vi "HandleObservationSync.vi"(8 "error in (no error)":errorcluster, 11 "S4GUI in":refnum<class "S4GUI.lvclass">) -> (0 "error out":errorcluster, 3 "S4GUI out":refnum<class "S4GUI.lvclass">)   [LabVIEW 2018, in "S4GUI.lvclass"] (continued)
              n761 = call-dynamic "Write Channel.vi"("error in (no error)"=w2070, "Channel.lvclass"=w2072, "Acquisition in"=w2077) -> ("error out"=w2075:errorcluster, "Acquisition out"=w2076:refnum<class "Acquisition.lvclass">)  [unwired: 7 in]
            }
          }
          n762 = call-dynamic "Write AcquisitionA.vi"("error in (no error)"=w1986, "Acquisition.lvclass"=w1988, "S4ACS_GUI in"=w1987) -> ("error out"=w1982:errorcluster, "S4ACS_GUI out"=w1981:refnum<class "S4GUI.lvclass">)  [unwired: 7 in]
          n763 = call "Read AcquisitionB.vi"("error in (no error)"=w1982, "S4ACS_GUI in"=w1981) -> ("error out"=w1964:errorcluster, "Acquisition.lvclass"=w1967:refnum<class "Acquisition.lvclass">, "S4ACS_GUI out"=w1968:refnum<class "S4GUI.lvclass">)  [unwired: 7 in]
          n764 = call "Read connection.vi"("error in (no error)"=w1964, "Server in"=w1967) -> ("error out"=w1963:errorcluster, "connection"=w1965:bool, "Server out"=w1966:refnum<class "Acquisition.lvclass">)  [unwired: 7 in]
          n765 = case shown="True" w1965 {
            tunnel: w1966 -> [w2045 w2061]
            tunnel: w1963 -> [w2044 w2060]
            tunnel: [w2045 w2058] -> w1962
            tunnel: [w2044 w2057] -> w1961
            tunnel: [0 ("State") w2047] -> w1931
            frame False {
            }
            frame True {
              n766 = call-dynamic "Read Channel.vi"("error in (no error)"=w2060, "Acquisition in"=w2061) -> ("error out"=w2056:errorcluster, "Channel.lvclass"=w2055:refnum<class "Channel.lvclass">, "Acquisition out"=w2059:refnum<class "Acquisition.lvclass">)  [unwired: 7 in]
              n767 = call-dynamic "Read State Machine.vi"("error in (no error)"=w2056, "Device in"=w2055) -> ("error out"=w2049:errorcluster, "State Machine.lvclass"=w2051:refnum<class "State Machine.lvclass">, "Device out"=w2053:refnum<class "Channel.lvclass">)  [unwired: 7 in]
              n768 = call-dynamic "Read State.vi"("error in (no error)"=w2049, "State Machine in"=w2051) -> ("error out"=w2048:errorcluster, "State"=w2047:i32, "State Machine out"=w2050:refnum<class "State Machine.lvclass">)  [unwired: 7 in]
              n769 = call-dynamic "Write State Machine.vi"("error in (no error)"=w2048, "State Machine.lvclass"=w2050, "Device in"=w2053) -> ("error out"=w2052:errorcluster, "Device out"=w2054:refnum<class "Channel.lvclass">)  [unwired: 7 in]
              n770 = call-dynamic "Write Channel.vi"("error in (no error)"=w2052, "Channel.lvclass"=w2054, "Acquisition in"=w2059) -> ("error out"=w2057:errorcluster, "Acquisition out"=w2058:refnum<class "Acquisition.lvclass">)  [unwired: 7 in]
            }
          }
          n771 = call "Write AcquisitionB.vi"("error in (no error)"=w1961, "Acquisition.lvclass"=w1962, "S4ACS_GUI in"=w1968) -> ("error out"=w1980:errorcluster, "S4ACS_GUI out"=w1979:refnum<class "S4GUI.lvclass">)  [unwired: 7 in]
          n772 = call-dynamic "Read AcquisitionC.vi"("error in (no error)"=w1980, "S4ACS_GUI in"=w1979) -> ("error out"=w1959:errorcluster, "Acquisition.lvclass"=w1960:refnum<class "Acquisition.lvclass">, "S4ACS_GUI out"=w1984:refnum<class "S4GUI.lvclass">)  [unwired: 7 in]
          n773 = call "Read connection.vi"("error in (no error)"=w1959, "Server in"=w1960) -> ("error out"=w1958:errorcluster, "connection"=w1956:bool, "Server out"=w1957:refnum<class "Acquisition.lvclass">)  [unwired: 7 in]
          n774 = case shown="True" w1956 {
            tunnel: w1957 -> [w2027 w2043]
            tunnel: w1958 -> [w2026 w2042]
            tunnel: [w2027 w2040] -> w1955
            tunnel: [w2026 w2039] -> w1954
            tunnel: [0 ("State") w2029] -> w1930
            frame False {
            }
            frame True {
              n775 = call-dynamic "Read Channel.vi"("error in (no error)"=w2042, "Acquisition in"=w2043) -> ("error out"=w2038:errorcluster, "Channel.lvclass"=w2037:refnum<class "Channel.lvclass">, "Acquisition out"=w2041:refnum<class "Acquisition.lvclass">)  [unwired: 7 in]
              n776 = call-dynamic "Read State Machine.vi"("error in (no error)"=w2038, "Device in"=w2037) -> ("error out"=w2031:errorcluster, "State Machine.lvclass"=w2033:refnum<class "State Machine.lvclass">, "Device out"=w2035:refnum<class "Channel.lvclass">)  [unwired: 7 in]
              n777 = call-dynamic "Read State.vi"("error in (no error)"=w2031, "State Machine in"=w2033) -> ("error out"=w2030:errorcluster, "State"=w2029:i32, "State Machine out"=w2032:refnum<class "State Machine.lvclass">)  [unwired: 7 in]
              n778 = call-dynamic "Write State Machine.vi"("error in (no error)"=w2030, "State Machine.lvclass"=w2032, "Device in"=w2035) -> ("error out"=w2034:errorcluster, "Device out"=w2036:refnum<class "Channel.lvclass">)  [unwired: 7 in]
              n779 = call-dynamic "Write Channel.vi"("error in (no error)"=w2034, "Channel.lvclass"=w2036, "Acquisition in"=w2041) -> ("error out"=w2039:errorcluster, "Acquisition out"=w2040:refnum<class "Acquisition.lvclass">)  [unwired: 7 in]
            }
          }
          n780 = call-dynamic "Write AcquisitionC.vi"("error in (no error)"=w1954, "Acquisition.lvclass"=w1955, "S4ACS_GUI in"=w1984) -> ("error out"=w1978:errorcluster, "S4ACS_GUI out"=w1977:refnum<class "S4GUI.lvclass">)  [unwired: 7 in]
          n781 = call-dynamic "Read AcquisitionD.vi"("error in (no error)"=w1978, "S4ACS_GUI in"=w1977) -> ("error out"=w1951:errorcluster, "Acquisition.lvclass"=w1953:refnum<class "Acquisition.lvclass">, "S4ACS_GUI out"=w1983:refnum<class "S4GUI.lvclass">)  [unwired: 7 in]
          n782 = call "Read connection.vi"("error in (no error)"=w1951, "Server in"=w1953) -> ("error out"=w1950:errorcluster, "connection"=w1949:bool, "Server out"=w1952:refnum<class "Acquisition.lvclass">)  [unwired: 7 in]
          n783 = case shown="True" w1949 {
            tunnel: w1952 -> [w2009 w2025]
            tunnel: w1950 -> [w2008 w2024]
            tunnel: [w2009 w2022] -> w1948
            tunnel: [w2008 w2021] -> w1947
            tunnel: [0 ("State") w2011] -> w1929
            frame False {
            }
            frame True {
              n784 = call-dynamic "Read Channel.vi"("error in (no error)"=w2024, "Acquisition in"=w2025) -> ("error out"=w2020:errorcluster, "Channel.lvclass"=w2019:refnum<class "Channel.lvclass">, "Acquisition out"=w2023:refnum<class "Acquisition.lvclass">)  [unwired: 7 in]
              n785 = call-dynamic "Read State Machine.vi"("error in (no error)"=w2020, "Device in"=w2019) -> ("error out"=w2013:errorcluster, "State Machine.lvclass"=w2015:refnum<class "State Machine.lvclass">, "Device out"=w2017:refnum<class "Channel.lvclass">)  [unwired: 7 in]
              n786 = call-dynamic "Read State.vi"("error in (no error)"=w2013, "State Machine in"=w2015) -> ("error out"=w2012:errorcluster, "State"=w2011:i32, "State Machine out"=w2014:refnum<class "State Machine.lvclass">)  [unwired: 7 in]
              n787 = call-dynamic "Write State Machine.vi"("error in (no error)"=w2012, "State Machine.lvclass"=w2014, "Device in"=w2017) -> ("error out"=w2016:errorcluster, "Device out"=w2018:refnum<class "Channel.lvclass">)  [unwired: 7 in]
              n788 = call-dynamic "Write Channel.vi"("error in (no error)"=w2016, "Channel.lvclass"=w2018, "Acquisition in"=w2023) -> ("error out"=w2021:errorcluster, "Acquisition out"=w2022:refnum<class "Acquisition.lvclass">)  [unwired: 7 in]
            }
          }
          n789 = call-dynamic "Write AcquisitionD.vi"("error in (no error)"=w1947, "Acquisition.lvclass"=w1948, "S4ACS_GUI in"=w1983) -> ("error out"=w1976:errorcluster, "S4ACS_GUI out"=w1941:refnum<class "S4GUI.lvclass">)  [unwired: 7 in]
          n790 = Equal?(x=w1933, y=w1932) -> (x = y?=w1937:bool)
          n791 = Equal?(x=w1942, y=w1932) -> (x = y?=w1946:bool)
          n792 = Equal?(x=w1933, y=w1931) -> (x = y?=w1936:bool)
          n793 = Equal?(x=w1942, y=w1931) -> (x = y?=w1945:bool)
          n794 = Equal?(x=w1933, y=w1930) -> (x = y?=w1935:bool)
          n795 = Equal?(x=w1942, y=w1930) -> (x = y?=w1944:bool)
          n796 = Equal?(x=w1933, y=w1929) -> (x = y?=w1934:bool)
          n797 = Equal?(x=w1942, y=w1929) -> (x = y?=w1943:bool)
          n798 = Compound Arithmetic op=ADD(w1932, w1931, w1930, w1929) -> (w1940:i32)
          n799 = Compound Arithmetic op=OR(w1937, w1936, w1935, w1934) -> (w1927:bool)
          n800 = Compound Arithmetic op=OR(w1946, w1945, w1944, w1943) -> (w1928:bool)
          n801 = Build Array(w1928, w1927) -> (w1926:bool[])
          n802 = Boolean Array To Number(Boolean array=w1926) -> (number=w1925:u32)
          n803 = case shown="0, Default" w1925 {
            tunnel: w1941 -> [w1991 w1999 w2003 w2007]
            tunnel: [w1990 w1998 w2002 w2006] -> w1938
            tunnel: w1940 -> [w1995 _ _ _]
            tunnel: w1939 -> [w1992 _ _ _]
            frame 0, Default {
              n804 = Equal To 0?(x=w1995) -> (x = 0?=w1994:bool)
              n805 = Select(t=u32 360, s=w1994, f=w1992) -> (s? t:f=w1989:u32)
              n806 = Bundle By Name(cluster=w1991, "Obs_state"=w1989) -> (w1990:refnum<class "S4GUI.lvclass">)
            }
            frame 1 {
              n807 = Bundle By Name(cluster=w1999, "Obs_state"=u32 1, "Error Msg"="ERROR: Some channel initialization failed. S4GUI:HandleObservationSync.vi state 272.") -> (w1998:refnum<class "S4GUI.lvclass">)
            }
            frame 2 {
              n808 = Bundle By Name(cluster=w2003, "Obs_state"=u32 1, "Error Msg"="ERROR: Some channel with invalid Exposition Time. S4GUI:HandleObservationSync.vi state 272.") -> (w2002:refnum<class "S4GUI.lvclass">)
            }
            frame 3 {
              n809 = Bundle By Name(cluster=w2007, "Obs_state"=u32 1, "Error Msg"="ERROR: Invalid configuration in the channels. S4GUI:HandleObservationSync.vi state 272.") -> (w2006:refnum<class "S4GUI.lvclass">)
            }
          }
        }
        frame 299 {
          # "Verifcando iniciação dos CICLO:"
          # "T= todos os canais ativos estão zerados."
          # "Exemplo de erro em \"Cycles_done\":\nchA; cycles_done=0; CCD_STATUS=ACTIVE;                                           Seqs_done=15;\nchA; cycles_done=0; CCD_STATUS=IDLE;                                                Seqs_done=16;   =>mudança de seq. com mesmo ciclo\nchA; cycles_done=1; CCD_STATUS=WAITING_EXPOSE_COMMAND; Seqs_done=0;\n\nchB; cycles_done=0; CCD_STATUS=ACTIVE;                                           Seqs_done=15;\nchB; cycles_done=1; CCD_STATUS=WAITING_EXPOSE_COMMAND; Seqs_done=0;     => mudança de seq com novo ciclo"
          # "T=canais receberam STOP"
          # "T= Todos os canais ativos no mesmo ciclo;\nF= Canais em ciclo diferente."
          # "Todos os CYCLES_DONE \nestão zerados?\nSe sim, vai para 327."
          # "Exemplo:\nSET #CYCLES 3\nSET #SEQ 4\ntotal de sequencias: 3 x 4 = 12\n\nseq.        CYCLES_DONE           SEQS_DONE\n1a.                     0                                 0\n2a.                     0                                 1 \n3a.                     0                                 2 \n4a.                     0                                 3 \n                          1                                 4\n5a.                     1                                 0 \n6a.                     1                                 1 \n7a.                     1                                 2 \n8a.                     1                                 3 \n                          2                                 4\n9a.                     2                                 0 \n10a.                   2                                 1 \n11a.                   2                                 2 \n12a.                   2                                 3 \n\nfim                    3                                 4"
          n810 = call-dynamic "Read AcquisitionA.vi"("error in (no error)"=w2132, "S4ACS_GUI in"=w2098) -> ("error out"=w2113:errorcluster, "Acquisition.lvclass"=w2114:refnum<class "Acquisition.lvclass">, "S4ACS_GUI out"=w2134:refnum<class "S4GUI.lvclass">)  [unwired: 7 in]
          n811 = call-dynamic "Read enabled.vi"("error in (no error)"=w2113, "Server in"=w2114) -> ("error out"=w2112:errorcluster, "enabled"=w2093:bool, "Server out"=w2111:refnum<class "Acquisition.lvclass">)  [unwired: 7 in]
          n812 = case shown="True" w2093 {
            tunnel: w2112 -> [w2224 w2240]
            tunnel: [w2225 w2238] -> w2135
            tunnel: [w2224 w2237] -> w2133
            tunnel: [u32 0 ("SequesDone") w2236] -> _
            tunnel: w2111 -> [w2225 w2235]
            tunnel: [TRUE w2234] -> w2097
            tunnel: [FALSE ("stopping") w2227] -> w2089
            frame False {
            }
            frame True {
              # "CYCLES_DONE = 0 ?"
              n813 = call-dynamic "Read Channel.vi"("error in (no error)"=w2240, "Acquisition in"=w2235) -> ("error out"=w2232:errorcluster, "Channel.lvclass"=w2233:refnum<class "Channel.lvclass">, "Acquisition out"=w2239:refnum<class "Acquisition.lvclass">)  [unwired: 7 in]
              n814 = call-dynamic "Read CyclesDone.vi"("error in (no error)"=w2232, "Channel in"=w2233) -> ("error out"=w2230:errorcluster, "CyclesDone"=w2236:u32, "Channel out"=w2231:refnum<class "Channel.lvclass">)  [unwired: 7 in]
              n815 = Equal?(x=w2236, y=u32 0) -> (x = y?=w2234:bool)
              n816 = call-dynamic "Read stopping.vi"("error in (no error)"=w2230, "Channel in"=w2231) -> ("error out"=w2229:errorcluster, "stopping"=w2227:bool, "Channel out"=w2228:refnum<class "Channel.lvclass">)  [unwired: 7 in]
              n817 = call-dynamic "Write Channel.vi"("error in (no error)"=w2229, "Channel.lvclass"=w2228, "Acquisition in"=w2239) -> ("error out"=w2237:errorcluster, "Acquisition out"=w2238:refnum<class "Acquisition.lvclass">)  [unwired: 7 in]
            }
          }
          n818 = call-dynamic "Write AcquisitionA.vi"("error in (no error)"=w2133, "Acquisition.lvclass"=w2135, "S4ACS_GUI in"=w2134) -> ("error out"=w2130:errorcluster, "S4ACS_GUI out"=w2129:refnum<class "S4GUI.lvclass">)  [unwired: 7 in]
          n819 = call "Read AcquisitionB.vi"("error in (no error)"=w2130, "S4ACS_GUI in"=w2129) -> ("error out"=w2107:errorcluster, "Acquisition.lvclass"=w2110:refnum<class "Acquisition.lvclass">, "S4ACS_GUI out"=w2131:refnum<class "S4GUI.lvclass">)  [unwired: 7 in]
          n820 = call-dynamic "Read enabled.vi"("error in (no error)"=w2107, "Server in"=w2110) -> ("error out"=w2108:errorcluster, "enabled"=w2092:bool, "Server out"=w2109:refnum<class "Acquisition.lvclass">)  [unwired: 7 in]
          n821 = case shown="True" w2092 {
            tunnel: w2108 -> [w2204 w2220]
            tunnel: w2109 -> [w2205 w2219]
            tunnel: [u32 0 ("SequesDone") w2214] -> _
            tunnel: [w2204 w2218] -> w2128
            tunnel: [w2205 w2217] -> w2127
            tunnel: [TRUE w2213] -> w2096
            tunnel: [FALSE ("stopping") w2207] -> w2088
            frame False {
            }
            frame True {
              n822 = call-dynamic "Read Channel.vi"("error in (no error)"=w2220, "Acquisition in"=w2219) -> ("error out"=w2211:errorcluster, "Channel.lvclass"=w2212:refnum<class "Channel.lvclass">, "Acquisition out"=w2215:refnum<class "Acquisition.lvclass">)  [unwired: 7 in]
              n823 = call-dynamic "Read CyclesDone.vi"("error in (no error)"=w2211, "Channel in"=w2212) -> ("error out"=w2209:errorcluster, "CyclesDone"=w2214:u32, "Channel out"=w2216:refnum<class "Channel.lvclass">)  [unwired: 7 in]
              n824 = Equal?(x=w2214, y=u32 0) -> (x = y?=w2213:bool)
              n825 = call-dynamic "Read stopping.vi"("error in (no error)"=w2209, "Channel in"=w2216) -> ("error out"=w2208:errorcluster, "stopping"=w2207:bool, "Channel out"=w2210:refnum<class "Channel.lvclass">)  [unwired: 7 in]
              n826 = call-dynamic "Write Channel.vi"("error in (no error)"=w2208, "Channel.lvclass"=w2210, "Acquisition in"=w2215) -> ("error out"=w2218:errorcluster, "Acquisition out"=w2217:refnum<class "Acquisition.lvclass">)  [unwired: 7 in]
            }
          }
          n827 = call "Write AcquisitionB.vi"("error in (no error)"=w2128, "Acquisition.lvclass"=w2127, "S4ACS_GUI in"=w2131) -> ("error out"=w2120:errorcluster, "S4ACS_GUI out"=w2119:refnum<class "S4GUI.lvclass">)  [unwired: 7 in]
          n828 = call-dynamic "Read AcquisitionC.vi"("error in (no error)"=w2120, "S4ACS_GUI in"=w2119) -> ("error out"=w2104:errorcluster, "Acquisition.lvclass"=w2106:refnum<class "Acquisition.lvclass">, "S4ACS_GUI out"=w2122:refnum<class "S4GUI.lvclass">)  [unwired: 7 in]
          n829 = call-dynamic "Read enabled.vi"("error in (no error)"=w2104, "Server in"=w2106) -> ("error out"=w2103:errorcluster, "enabled"=w2091:bool, "Server out"=w2105:refnum<class "Acquisition.lvclass">)  [unwired: 7 in]
          n830 = case shown="True" w2091 {
            tunnel: [w2184 w2200] -> w2123
            tunnel: [w2185 w2199] -> w2121
            tunnel: w2103 -> [w2184 w2196]
            tunnel: w2105 -> [w2185 w2197]
            tunnel: [u32 0 ("SequesDone") w2195] -> _
            tunnel: [TRUE w2194] -> w2095
            tunnel: [FALSE ("stopping") w2187] -> w2087
            frame False {
            }
            frame True {
              n831 = call-dynamic "Read Channel.vi"("error in (no error)"=w2196, "Acquisition in"=w2197) -> ("error out"=w2191:errorcluster, "Channel.lvclass"=w2192:refnum<class "Channel.lvclass">, "Acquisition out"=w2198:refnum<class "Acquisition.lvclass">)  [unwired: 7 in]
              n832 = call-dynamic "Read CyclesDone.vi"("error in (no error)"=w2191, "Channel in"=w2192) -> ("error out"=w2189:errorcluster, "CyclesDone"=w2195:u32, "Channel out"=w2193:refnum<class "Channel.lvclass">)  [unwired: 7 in]
              n833 = Equal?(x=w2195, y=u32 0) -> (x = y?=w2194:bool)
              n834 = call-dynamic "Read stopping.vi"("error in (no error)"=w2189, "Channel in"=w2193) -> ("error out"=w2188:errorcluster, "stopping"=w2187:bool, "Channel out"=w2190:refnum<class "Channel.lvclass">)  [unwired: 7 in]
              n835 = call-dynamic "Write Channel.vi"("error in (no error)"=w2188, "Channel.lvclass"=w2190, "Acquisition in"=w2198) -> ("error out"=w2200:errorcluster, "Acquisition out"=w2199:refnum<class "Acquisition.lvclass">)  [unwired: 7 in]
            }
          }
          n836 = call-dynamic "Write AcquisitionC.vi"("error in (no error)"=w2123, "Acquisition.lvclass"=w2121, "S4ACS_GUI in"=w2122) -> ("error out"=w2117:errorcluster, "S4ACS_GUI out"=w2118:refnum<class "S4GUI.lvclass">)  [unwired: 7 in]
          n837 = call-dynamic "Read AcquisitionD.vi"("error in (no error)"=w2117, "S4ACS_GUI in"=w2118) -> ("error out"=w2100:errorcluster, "Acquisition.lvclass"=w2102:refnum<class "Acquisition.lvclass">, "S4ACS_GUI out"=w2124:refnum<class "S4GUI.lvclass">)  [unwired: 7 in]
          n838 = call-dynamic "Read enabled.vi"("error in (no error)"=w2100, "Server in"=w2102) -> ("error out"=w2099:errorcluster, "enabled"=w2090:bool, "Server out"=w2101:refnum<class "Acquisition.lvclass">)  [unwired: 7 in]
          n839 = case shown="True" w2090 {
            tunnel: [w2165 w2180] -> w2126
            tunnel: [w2164 w2179] -> w2125
            tunnel: w2101 -> [w2165 w2178]
            tunnel: w2099 -> [w2164 w2177]
            tunnel: [u32 0 ("SequesDone") w2175] -> _
            tunnel: [TRUE w2174] -> w2094
            tunnel: [FALSE ("stopping") w2167] -> w2086
            frame False {
            }
            frame True {
              n840 = call-dynamic "Read Channel.vi"("error in (no error)"=w2177, "Acquisition in"=w2178) -> ("error out"=w2171:errorcluster, "Channel.lvclass"=w2172:refnum<class "Channel.lvclass">, "Acquisition out"=w2176:refnum<class "Acquisition.lvclass">)  [unwired: 7 in]
              n841 = call-dynamic "Read CyclesDone.vi"("error in (no error)"=w2171, "Channel in"=w2172) -> ("error out"=w2169:errorcluster, "CyclesDone"=w2175:u32, "Channel out"=w2173:refnum<class "Channel.lvclass">)  [unwired: 7 in]
              n842 = Equal?(x=w2175, y=u32 0) -> (x = y?=w2174:bool)
              n843 = call-dynamic "Read stopping.vi"("error in (no error)"=w2169, "Channel in"=w2173) -> ("error out"=w2168:errorcluster, "stopping"=w2167:bool, "Channel out"=w2170:refnum<class "Channel.lvclass">)  [unwired: 7 in]
              n844 = call-dynamic "Write Channel.vi"("error in (no error)"=w2168, "Channel.lvclass"=w2170, "Acquisition in"=w2176) -> ("error out"=w2179:errorcluster, "Acquisition out"=w2180:refnum<class "Acquisition.lvclass">)  [unwired: 7 in]
            }
          }
          n845 = Compound Arithmetic op=AND(w2097, w2096, w2095, w2094) -> (w2083:bool)
          n846 = Compound Arithmetic op=OR(w2089, w2088, w2087, w2086) -> (w2085:bool)
          n847 = call-dynamic "Write AcquisitionD.vi"("error in (no error)"=w2125, "Acquisition.lvclass"=w2126, "S4ACS_GUI in"=w2124) -> ("error out"=w2115:errorcluster, "S4ACS_GUI out"=w2116:refnum<class "S4GUI.lvclass">)  [unwired: 7 in]
          n848 = case shown="True" w2083 {
            tunnel: w2116 -> [w2146 w2157]
            tunnel: [w2145 w2156] -> w2084
            tunnel: w2085 -> [_ w2155]
            tunnel: w2082 -> [_ w2152]
            frame False {
              # "Esperando todos os canais habilitados mudarem de cyclesDone.\nE verificando a maior duracao de cubo entre os canais."
              n849 = local read "time307"() -> (w2144:u32)
              n850 = Tick Count (ms)() -> (millisecond timer value=w2143:u32)
              n851 = Subtract(x=w2143, y=w2144) -> (x-y=w2139:u32)
              n852 = call-dynamic "GetGreatestCube.vi"("S4GUI in"=w2146) -> ("S4GUI out"=w2141:refnum<class "S4GUI.lvclass">, "greatest (ms)"=w2137:dbl)  [unwired: 8 in, 1 out]
              n853 = To Double Precision Float(number=w2139) -> (double precision float=w2142:dbl)
              n854 = Add(x=1000.0 ("y"), y=w2137) -> (x+y=w2136:dbl)
              n855 = Less?(x=w2136, y=w2142) -> (x < y?=w2140:bool)
              n856 = case shown="False" w2140 {
                tunnel: w2141 -> [w2147 w2151]
                tunnel: [w2147 w2150] -> w2145
                frame False {
                }
                frame True {
                  n857 = Bundle By Name(cluster=w2151, "Obs_state"=u32 1, "Error Msg"="ERROR: Cycles_Done reseting timeout. - HandleObservationSync.vi state 299.") -> (w2150:refnum<class "S4GUI.lvclass">)
                }
              }
            }
            frame True {
              # "STOP?"
              n858 = case shown="False" w2155 {
                tunnel: [w2158 u32 0] -> w2154
                tunnel: w2152 -> [w2159 _]
                frame False {
                  n859 = Increment(x=w2159) -> (x+1=w2158:u32)
                }
                frame True {
                }
              }
              n860 = Bundle By Name(cluster=w2157, "Obs_state"=w2154, "cyclesDone"=u32 0) -> (w2156:refnum<class "S4GUI.lvclass">)
            }
          }
        }
        frame 300 {
          # "Verifica se é modo fotometria ou polarimetria:\nTrue = polarimetria (esatdo 301)\nFalse = fotometria (estado 321)"
          n861 = flat-sequence {
            tunnel: w2245 -> [w2258]
            tunnel: [w2258] -> w2244
            frame #0 {
              n862 = local read "time3"() -> (w2260:u32)
              n863 = local read "time4"() -> (w2257:u32)
              n864 = Tick Count (ms)() -> (millisecond timer value=w2256:u32)
              n865 = Subtract(x=w2257, y=w2260) -> (x-y=→"delay 3-4":u32)
              n866 = local write "time1"(w2256) -> ()
            }
          }
          n867 = call "Read Instrument.lvclass.vi"("error in (no error)"=w2244, "S4ACS_GUI in"=w2255) -> ("error out"=w2250:errorcluster, "Instrument.lvclass"=w2251:refnum<class "Instrument.lvclass">, "S4ACS_GUI out"=w2249:refnum<class "S4GUI.lvclass">)  [unwired: 7 in]
          n868 = call-dynamic "Read mode.vi"("error in (no error)"=w2250, "Instrument in"=w2251) -> ("error out"=w2246:errorcluster, "mode"=w2248:bool)  [unwired: 7 in, 1 out]
          n869 = Select(t=u32 301, s=w2248, f=u32 321 ("t")) -> (s? t:f=w2253:u32)
          n870 = Bundle By Name(cluster=w2249, "Obs_state"=w2253, "cyclesDone"=u32 0, "sequesDone"=u32 0, "seqAtual"=u32 0) -> (w2254:refnum<class "S4GUI.lvclass">)
        }
        frame 301 {
          # "Configurando para ACS esperar comando EXPOSE"
          n871 = call-dynamic "Read AcquisitionA.vi"("error in (no error)"=w2323, "S4ACS_GUI in"=w2324) -> ("error out"=w2278:errorcluster, "Acquisition.lvclass"=w2279:refnum<class "Acquisition.lvclass">, "S4ACS_GUI out"=w2326:refnum<class "S4GUI.lvclass">)  [unwired: 7 in]
          n872 = call-dynamic "Read enabled.vi"("error in (no error)"=w2278, "Server in"=w2279) -> ("error out"=w2277:errorcluster, "enabled"=w2264:bool, "Server out"=w2280:refnum<class "Acquisition.lvclass">)  [unwired: 7 in]
          n873 = call "Read connection.vi"("error in (no error)"=w2277, "Server in"=w2280) -> ("error out"=w2303:errorcluster, "connection"=w2287:bool, "Server out"=w2304:refnum<class "Acquisition.lvclass">)  [unwired: 7 in]
          n874 = And(x=w2287, y=w2264) -> (x .and. y?=w2288:bool)
          n875 = case shown="True" w2288 {
            tunnel: w2304 -> [w2441 w2460]
            tunnel: w2303 -> [w2440 w2459]
            tunnel: [w2441 w2457] -> w2327
            tunnel: [w2440 w2456] -> w2325
            tunnel: [w2437 u32 0 ("New_State")] -> w2293
            tunnel: w2264 -> [w2436 _]
            frame False {
              n876 = Select(t=u32 1, s=w2436, f=u32 0) -> (s? t:f=w2437:u32)
            }
            frame True {
              n877 = call-dynamic "Read Channel.vi"("error in (no error)"=w2459, "Acquisition in"=w2460) -> ("error out"=w2443:errorcluster, "Channel.lvclass"=w2446:refnum<class "Channel.lvclass">, "Acquisition out"=w2458:refnum<class "Acquisition.lvclass">)  [unwired: 7 in]
              n878 = call-dynamic "Write wait_expose.vi"("error in (no error)"=w2443, "wait_expose"=TRUE, "Channel in"=w2446) -> ("error out"=w2442:errorcluster, "Channel out"=w2445:refnum<class "Channel.lvclass">)  [unwired: 7 in]
              n879 = call-dynamic "Read State Machine.vi"("error in (no error)"=w2442, "Device in"=w2445) -> ("error out"=w2453:errorcluster, "State Machine.lvclass"=w2455:refnum<class "State Machine.lvclass">, "Device out"=w2451:refnum<class "Channel.lvclass">)  [unwired: 7 in]
              n880 = call "Next State.vi"("error in (no error)"=w2453, "New_State"=40, "State Machine in"=w2455) -> ("error out"=w2448:errorcluster, "State Machine out"=w2449:refnum<class "State Machine.lvclass">)  [unwired: 7 in]
              n881 = call-dynamic "Write State Machine.vi"("error in (no error)"=w2448, "State Machine.lvclass"=w2449, "Device in"=w2451) -> ("error out"=w2450:errorcluster, "Device out"=w2452:refnum<class "Channel.lvclass">)  [unwired: 7 in]
              n882 = call-dynamic "Write Channel.vi"("error in (no error)"=w2450, "Channel.lvclass"=w2452, "Acquisition in"=w2458) -> ("error out"=w2456:errorcluster, "Acquisition out"=w2457:refnum<class "Acquisition.lvclass">)  [unwired: 7 in]
            }
          }
          n883 = call-dynamic "Write AcquisitionA.vi"("error in (no error)"=w2325, "Acquisition.lvclass"=w2327, "S4ACS_GUI in"=w2326) -> ("error out"=w2320:errorcluster, "S4ACS_GUI out"=w2321:refnum<class "S4GUI.lvclass">)  [unwired: 7 in]
          n884 = call "Read AcquisitionB.vi"("error in (no error)"=w2320, "S4ACS_GUI in"=w2321) -> ("error out"=w2274:errorcluster, "Acquisition.lvclass"=w2276:refnum<class "Acquisition.lvclass">, "S4ACS_GUI out"=w2318:refnum<class "S4GUI.lvclass">)  [unwired: 7 in]
          n885 = call-dynamic "Read enabled.vi"("error in (no error)"=w2274, "Server in"=w2276) -> ("error out"=w2273:errorcluster, "enabled"=w2263:bool, "Server out"=w2275:refnum<class "Acquisition.lvclass">)  [unwired: 7 in]
          n886 = call "Read connection.vi"("error in (no error)"=w2273, "Server in"=w2275) -> ("error out"=w2301:errorcluster, "connection"=w2285:bool, "Server out"=w2302:refnum<class "Acquisition.lvclass">)  [unwired: 7 in]
          n887 = And(x=w2285, y=w2263) -> (x .and. y?=w2286:bool)
          n888 = case shown="False" w2286 {
            tunnel: w2302 -> [w2416 w2435]
            tunnel: w2301 -> [w2415 w2434]
            tunnel: [w2416 w2432] -> w2319
            tunnel: [w2415 w2431] -> w2317
            tunnel: [w2412 u32 0 ("New_State")] -> w2292
            tunnel: w2263 -> [w2411 _]
            frame False {
              n889 = Select(t=u32 2, s=w2411, f=u32 0) -> (s? t:f=w2412:u32)
            }
            frame True {
              n890 = call-dynamic "Read Channel.vi"("error in (no error)"=w2434, "Acquisition in"=w2435) -> ("error out"=w2418:errorcluster, "Channel.lvclass"=w2420:refnum<class "Channel.lvclass">, "Acquisition out"=w2433:refnum<class "Acquisition.lvclass">)  [unwired: 7 in]
              n891 = call-dynamic "Write wait_expose.vi"("error in (no error)"=w2418, "wait_expose"=TRUE, "Channel in"=w2420) -> ("error out"=w2417:errorcluster, "Channel out"=w2419:refnum<class "Channel.lvclass">)  [unwired: 7 in]
              n892 = call-dynamic "Read State Machine.vi"("error in (no error)"=w2417, "Device in"=w2419) -> ("error out"=w2428:errorcluster, "State Machine.lvclass"=w2430:refnum<class "State Machine.lvclass">, "Device out"=w2426:refnum<class "Channel.lvclass">)  [unwired: 7 in]
              n893 = call "Next State.vi"("error in (no error)"=w2428, "New_State"=40, "State Machine in"=w2430) -> ("error out"=w2423:errorcluster, "State Machine out"=w2424:refnum<class "State Machine.lvclass">)  [unwired: 7 in]
              n894 = call-dynamic "Write State Machine.vi"("error in (no error)"=w2423, "State Machine.lvclass"=w2424, "Device in"=w2426) -> ("error out"=w2425:errorcluster, "Device out"=w2427:refnum<class "Channel.lvclass">)  [unwired: 7 in]
              n895 = call-dynamic "Write Channel.vi"("error in (no error)"=w2425, "Channel.lvclass"=w2427, "Acquisition in"=w2433) -> ("error out"=w2431:errorcluster, "Acquisition out"=w2432:refnum<class "Acquisition.lvclass">)  [unwired: 7 in]
            }
          }
          n896 = call "Write AcquisitionB.vi"("error in (no error)"=w2317, "Acquisition.lvclass"=w2319, "S4ACS_GUI in"=w2318) -> ("error out"=w2313:errorcluster, "S4ACS_GUI out"=w2312:refnum<class "S4GUI.lvclass">)  [unwired: 7 in]
          n897 = call-dynamic "Read AcquisitionC.vi"("error in (no error)"=w2313, "S4ACS_GUI in"=w2312) -> ("error out"=w2270:errorcluster, "Acquisition.lvclass"=w2272:refnum<class "Acquisition.lvclass">, "S4ACS_GUI out"=w2315:refnum<class "S4GUI.lvclass">)  [unwired: 7 in]
          n898 = call-dynamic "Read enabled.vi"("error in (no error)"=w2270, "Server in"=w2272) -> ("error out"=w2269:errorcluster, "enabled"=w2262:bool, "Server out"=w2271:refnum<class "Acquisition.lvclass">)  [unwired: 7 in]
          n899 = call "Read connection.vi"("error in (no error)"=w2269, "Server in"=w2271) -> ("error out"=w2299:errorcluster, "connection"=w2282:bool, "Server out"=w2300:refnum<class "Acquisition.lvclass">)  [unwired: 7 in]
          n900 = And(x=w2282, y=w2262) -> (x .and. y?=w2284:bool)
          n901 = case shown="True" w2284 {
            tunnel: [w2390 w2404] -> w2316
            tunnel: [w2391 w2403] -> w2314
            tunnel: w2300 -> [w2391 w2401]
            tunnel: w2299 -> [w2390 w2400]
            tunnel: [w2387 u32 0 ("New_State")] -> w2291
            tunnel: w2262 -> [w2386 _]
            frame False {
              n902 = Select(t=u32 4, s=w2386, f=u32 0) -> (s? t:f=w2387:u32)
            }
            frame True {
              n903 = call-dynamic "Read Channel.vi"("error in (no error)"=w2400, "Acquisition in"=w2401) -> ("error out"=w2393:errorcluster, "Channel.lvclass"=w2395:refnum<class "Channel.lvclass">, "Acquisition out"=w2402:refnum<class "Acquisition.lvclass">)  [unwired: 7 in]
              n904 = call-dynamic "Write wait_expose.vi"("error in (no error)"=w2393, "wait_expose"=TRUE, "Channel in"=w2395) -> ("error out"=w2392:errorcluster, "Channel out"=w2394:refnum<class "Channel.lvclass">)  [unwired: 7 in]
              n905 = call-dynamic "Read State Machine.vi"("error in (no error)"=w2392, "Device in"=w2394) -> ("error out"=w2407:errorcluster, "State Machine.lvclass"=w2405:refnum<class "State Machine.lvclass">, "Device out"=w2409:refnum<class "Channel.lvclass">)  [unwired: 7 in]
              n906 = call "Next State.vi"("error in (no error)"=w2407, "New_State"=40, "State Machine in"=w2405) -> ("error out"=w2399:errorcluster, "State Machine out"=w2398:refnum<class "State Machine.lvclass">)  [unwired: 7 in]
              n907 = call-dynamic "Write State Machine.vi"("error in (no error)"=w2399, "State Machine.lvclass"=w2398, "Device in"=w2409) -> ("error out"=w2410:errorcluster, "Device out"=w2408:refnum<class "Channel.lvclass">)  [unwired: 7 in]
              n908 = call-dynamic "Write Channel.vi"("error in (no error)"=w2410, "Channel.lvclass"=w2408, "Acquisition in"=w2402) -> ("error out"=w2404:errorcluster, "Acquisition out"=w2403:refnum<class "Acquisition.lvclass">)  [unwired: 7 in]
            }
          }
          n909 = call-dynamic "Write AcquisitionC.vi"("error in (no error)"=w2316, "Acquisition.lvclass"=w2314, "S4ACS_GUI in"=w2315) -> ("error out"=w2310:errorcluster, "S4ACS_GUI out"=w2309:refnum<class "S4GUI.lvclass">)  [unwired: 7 in]
          n910 = call-dynamic "Read AcquisitionD.vi"("error in (no error)"=w2310, "S4ACS_GUI in"=w2309) -> ("error out"=w2266:errorcluster, "Acquisition.lvclass"=w2268:refnum<class "Acquisition.lvclass">, "S4ACS_GUI out"=w2308:refnum<class "S4GUI.lvclass">)  [unwired: 7 in]
          n911 = call-dynamic "Read enabled.vi"("error in (no error)"=w2266, "Server in"=w2268) -> ("error out"=w2265:errorcluster, "enabled"=w2261:bool, "Server out"=w2267:refnum<class "Acquisition.lvclass">)  [unwired: 7 in]
          n912 = call "Read connection.vi"("error in (no error)"=w2265, "Server in"=w2267) -> ("error out"=w2297:errorcluster, "connection"=w2281:bool, "Server out"=w2298:refnum<class "Acquisition.lvclass">)  [unwired: 7 in]
          n913 = And(x=w2281, y=w2261) -> (x .and. y?=w2283:bool)
          n914 = case shown="True" w2283 {
            tunnel: w2297 -> [w2365 w2385]
            tunnel: [w2365 w2384] -> w2311
            tunnel: w2298 -> [w2366 w2377]
            tunnel: [w2366 w2375] -> w2307
            tunnel: [w2362 u32 0 ("New_State")] -> w2290
            tunnel: w2261 -> [w2361 _]
            frame False {
              n915 = Select(t=u32 8, s=w2361, f=u32 0) -> (s? t:f=w2362:u32)
            }
            frame True {
              n916 = call-dynamic "Read Channel.vi"("error in (no error)"=w2385, "Acquisition in"=w2377) -> ("error out"=w2367:errorcluster, "Channel.lvclass"=w2370:refnum<class "Channel.lvclass">, "Acquisition out"=w2376:refnum<class "Acquisition.lvclass">)  [unwired: 7 in]
              n917 = call-dynamic "Write wait_expose.vi"("error in (no error)"=w2367, "wait_expose"=TRUE, "Channel in"=w2370) -> ("error out"=w2368:errorcluster, "Channel out"=w2369:refnum<class "Channel.lvclass">)  [unwired: 7 in]
              n918 = call-dynamic "Read State Machine.vi"("error in (no error)"=w2368, "Device in"=w2369) -> ("error out"=w2381:errorcluster, "State Machine.lvclass"=w2383:refnum<class "State Machine.lvclass">, "Device out"=w2379:refnum<class "Channel.lvclass">)  [unwired: 7 in]
              n919 = call "Next State.vi"("error in (no error)"=w2381, "New_State"=40, "State Machine in"=w2383) -> ("error out"=w2373:errorcluster, "State Machine out"=w2374:refnum<class "State Machine.lvclass">)  [unwired: 7 in]
              n920 = call-dynamic "Write State Machine.vi"("error in (no error)"=w2373, "State Machine.lvclass"=w2374, "Device in"=w2379) -> ("error out"=w2378:errorcluster, "Device out"=w2380:refnum<class "Channel.lvclass">)  [unwired: 7 in]
              n921 = call-dynamic "Write Channel.vi"("error in (no error)"=w2378, "Channel.lvclass"=w2380, "Acquisition in"=w2376) -> ("error out"=w2384:errorcluster, "Acquisition out"=w2375:refnum<class "Acquisition.lvclass">)  [unwired: 7 in]
            }
          }
          n922 = call-dynamic "Write AcquisitionD.vi"("error in (no error)"=w2311, "Acquisition.lvclass"=w2307, "S4ACS_GUI in"=w2308) -> ("error out"=w2306:errorcluster, "S4ACS_GUI out"=w2305:refnum<class "S4GUI.lvclass">)  [unwired: 7 in]
          n923 = Compound Arithmetic op=ADD(w2293, w2292, w2291, w2290) -> (w2294:u32)
          n924 = case shown="0, Default" w2294 {
            tunnel: w2289 -> [w2330 _ _ _ _ _ _ _ _ _ _ _ _ _ _ _]
            tunnel: [w2329 u32 1 ("Obs_state") u32 1 ("Obs_state") u32 1 ("Obs_state") u32 1 ("Obs_state") u32 1 ("Obs_state") u32 1 ("Obs_state") u32 1 ("Obs_state") u32 1 ("Obs_state") u32 1 ("Obs_state") u32 1 ("Obs_state") u32 1 ("Obs_state") u32 1 ("Obs_state") u32 1 ("Obs_state") u32 1 ("Obs_state") u32 1 ("Obs_state")] -> w2295
            tunnel: ["" ("Error Msg") "ERROR: Lost channel 1 connection... - HandleObservationSync.vi state 301" ("Error Msg") "ERROR: Lost channel 2 connection...- HandleObservationSync.vi state 301" ("Error Msg") "ERROR: Lost channels 1 and 2 connection...- HandleObservationSync.vi state 301" ("Error Msg") "ERROR: Lost channel 3 connection...- HandleObservationSync.vi state 301" ("Error Msg") "ERROR: Lost channels 1 and  3 connection...- HandleObservationSync.vi state 301" ("Error Msg") "ERROR:  Lost channels 2 and  3 connection...- HandleObservationSync.vi state 301" ("Error Msg") "ERROR:  Lost channels 1, 2 and  3 connection...- HandleObservationSync.vi state 301" ("Error Msg") "ERROR: Lost channel 4 connection...- HandleObservationSync.vi state 301" ("Error Msg") "ERROR:  Lost channels 1 and 4 connection...- HandleObservationSync.vi state 301" ("Error Msg") "ERROR:  Lost channels 2 and 4 connection...- HandleObservationSync.vi state 301" ("Error Msg") "ERROR: Lost channels 1, 2 and 4 connection...- HandleObservationSync.vi state 301" ("Error Msg") "ERROR: Lost channels 3 and 4 connection...- HandleObservationSync.vi state 301" ("Error Msg") "ERROR: Lost channels 1, 3 and 4 connection...- HandleObservationSync.vi state 301" ("Error Msg") "ERROR: Lost channels 2, 3 and 4 connection...- HandleObservationSync.vi state 301" ("Error Msg") "ERROR: Lost channels 1, 2, 3 and 4 connection...- HandleObservationSync.vi state 301" ("Error Msg")] -> w2296
            frame 0, Default {
              n925 = Increment(x=w2330) -> (x+1=w2329:u32)
            }
            frame 1 {
            }
            frame 2 {
            }
            frame 3 {
            }
            frame 4 {
            }
            frame 5 {
            }
            frame 6 {
            }
            frame 7 {
            }
            frame 8 {
            }
            frame 9 {
            }
            frame 10 {
            }
            frame 11 {
            }
            frame 12 {
            }
            frame 13 {
            }
            frame 14 {
            }
            frame 15 {
            }
          }
          n926 = Bundle By Name(cluster=w2305, "Obs_state"=w2295, "Error Msg"=w2296) -> (w2322:refnum<class "S4GUI.lvclass">)
        }
        frame 302 {
          # "Espera terminar o envio de WAIT EXPOSE COMMAND para todos os ACS."
          n927 = call-dynamic "VerifyAcqIdle.vi"("error in (no error)"=w2462, "S4GUI in"=w2461) -> ("error out"=w2467:errorcluster, "idle"=w2466:bool, "S4GUI out"=w2468:refnum<class "S4GUI.lvclass">)  [unwired: 6 in, 1 out]
          n928 = Increment(x=w2464) -> (x+1=w2463:u32)
          n929 = Select(t=w2463, s=w2466, f=w2464) -> (s? t:f=w2465:u32)
          n930 = Bundle By Name(cluster=w2468, "Obs_state"=w2465) -> (w2469:refnum<class "S4GUI.lvclass">)
        }
        frame 303 {
          n931 = flat-sequence {
            tunnel: w2475 -> [w2514]
            tunnel: [w2514] -> w2474
            frame #0 {
              n932 = Tick Count (ms)() -> (millisecond timer value=→"time1":u32)
            }
          }
          n933 = call "Read Instrument.lvclass.vi"("error in (no error)"=w2474, "S4ACS_GUI in"=w2510) -> ("error out"=w2512:errorcluster, "Instrument.lvclass"=w2513:refnum<class "Instrument.lvclass">, "S4ACS_GUI out"=w2471:refnum<class "S4GUI.lvclass">)  [unwired: 7 in]
          n934 = call "Read WPROT.vi"("error in (no error)"=w2512, "Instrument in"=w2513) -> ("error out"=w2503:errorcluster, "Opt_Selector.lvclass"=w2504:refnum<class "Opt_Selector.lvclass">, "Instrument out"=w2511:refnum<class "Instrument.lvclass">)  [unwired: 7 in]
          n935 = call-dynamic "getTargetPos.vi"("error in (no error)"=w2503, "Opt_Selector in"=w2504) -> ("error out"=w2502:errorcluster, "Target Pos"=w2482:u16, "Opt_Selector out"=w2501:refnum<class "Opt_Selector.lvclass">)  [unwired: 7 in]
          n936 = Unbundle By Name(w2471) -> ("seqAtual"=w2473:u32)
          n937 = Build Array(-1.0 ("element"), 0.0 ("element"), 22.5 ("element"), 45.0 ("element"), 67.5 ("element"), 90.0 ("element"), 112.5 ("element"), 135.0 ("element"), 157.5 ("element"), 180.0 ("element"), 202.5 ("element"), 225.0 ("element"), 247.5 ("element"), 270.0 ("element"), 292.5 ("element"), 315.0 ("element"), 337.5 ("element")) -> (w2494:dbl[])
          n938 = Index Array(array=w2494, index=w2482) -> (element=w2481:dbl)
          n939 = case shown="1..16" w2482 {
            selector: w2482 -> [_ w2548]
            tunnel: w2511 -> [w2524 w2536]
            tunnel: [w2524 w2536] -> w2477
            tunnel: [w2521 w2535] -> w2476
            tunnel: w2507 -> [_ w2550]
            tunnel: [u32 314 w2549] -> w2506
            tunnel: w2502 -> [w2522 w2544]
            tunnel: w2501 -> [w2523 w2543]
            tunnel: w2481 -> [_ w2538]
            tunnel: [w2519 w2537] -> w2478
            tunnel: [u32 0 w2526] -> w2472
            tunnel: w2473 -> [_ w2527]
            frame 0, Default {
              # "Terminou uma sequência.\nRecupera as posições em SEQ e desvia para 314 para verificar se há mais ciclos."
              # "Recupera a sequencia anterior para o caso \nde repetição da sequencia (sem precisar clicar \nnas posicoes desejadas novamente)."
              n940 = call-dynamic "Read sequencia_ant.vi"("error in (no error)"=w2522, "Opt_Selector in"=w2523) -> ("error out"=w2518:errorcluster, "sequencia_ant"=w2517:u16, "Opt_Selector out"=w2520:refnum<class "Opt_Selector.lvclass">)  [unwired: 7 in]
              n941 = call-dynamic "Write sequencia.vi"("error in (no error)"=w2518, "sequencia"=w2517, "Opt_Selector in"=w2520) -> ("error out"=w2521:errorcluster, "Opt_Selector out"=w2519:refnum<class "Opt_Selector.lvclass">)  [unwired: 7 in]
            }
            frame 1..16 {
              # "Inicia o Ticks com\nvalor do relogio atual"
              # "Espera até 40 x 0.25s (= 10s) para\nmecanismo entrar em READY"
              n942 = Number To Decimal String(number=w2548) -> (decimal integer string=w2547:string)  [unwired: 1 in]
              n943 = Concatenate Strings("WP" ("string"), w2547) -> (w2545:string)
              n944 = call "Write target name.vi"("error in (no error)"=w2544, "target name"=w2545, "Optics in"=w2543) -> ("error out"=w2541:errorcluster, "Optics out"=w2542:refnum<class "Opt_Selector.lvclass">)  [unwired: 7 in]
              n945 = call "Write target.vi"("error in (no error)"=w2541, "target"=w2538, "Optics in"=w2542) -> ("error out"=w2540:errorcluster, "Optics out"=w2539:refnum<class "Opt_Selector.lvclass">)  [unwired: 7 in]
              n946 = call-dynamic "Read State Machine.vi"("error in (no error)"=w2540, "Device in"=w2539) -> ("error out"=w2552:errorcluster, "State Machine.lvclass"=w2554:refnum<class "State Machine.lvclass">, "Device out"=w2551:refnum<class "Opt_Selector.lvclass">)  [unwired: 7 in]
              n947 = Increment(x=w2550) -> (x+1=w2549:u32)
              n948 = call "Next State.vi"("error in (no error)"=w2552, "New_State"=1, "State Machine in"=w2554) -> ("error out"=w2533:errorcluster, "State Machine out"=w2534:refnum<class "State Machine.lvclass">)  [unwired: 7 in]
              n949 = Increment(x=w2527) -> (x+1=w2526:u32)
              n950 = call-dynamic "Write Timer.vi"("error in (no error)"=w2533, "Timer"=u32 40, "State Machine in"=w2534) -> ("error out"=w2530:errorcluster, "State Machine out"=w2531:refnum<class "State Machine.lvclass">)  [unwired: 7 in]
              n951 = call-dynamic "Init Ticks2.vi"("error in (no error)"=w2530, "State Machine in"=w2531) -> ("error out"=w2529:errorcluster, "State Machine out"=w2528:refnum<class "State Machine.lvclass">)  [unwired: 8 in]
              n952 = call-dynamic "Write State Machine.vi"("error in (no error)"=w2529, "State Machine.lvclass"=w2528, "Device in"=w2551) -> ("error out"=w2535:errorcluster, "Device out"=w2537:refnum<class "Opt_Selector.lvclass">)  [unwired: 7 in]
            }
          }
          n953 = Bundle By Name(cluster=w2471, "seqAtual"=w2472) -> (w2470:refnum<class "S4GUI.lvclass">)
          n954 = call "Write WPROT.vi"("error in (no error)"=w2476, "Opt_Selector.lvclass"=w2478, "Instrument in"=w2477) -> ("error out"=w2480:errorcluster, "Instrument out"=w2479:refnum<class "Instrument.lvclass">)  [unwired: 7 in]
          n955 = call "Write Instrument.lvclass.vi"("error in (no error)"=w2480, "Instrument.lvclass"=w2479, "S4ACS_GUI in"=w2470) -> ("error out"=w2509:errorcluster, "S4ACS_GUI out"=w2508:refnum<class "S4GUI.lvclass">)  [unwired: 7 in]
          n956 = Bundle By Name(cluster=w2508, "Obs_state"=w2506) -> (w2505:refnum<class "S4GUI.lvclass">)
        }
        frame 304 {
          # "Para inserir Pausa antes do\nEXPOSE, ir para 305."
          # "Espera terminar o movimento da lamina para disparar a aquisição\ndos canais ativos.\n\nOV 20230424: Não precisa mais atualizar o valor de WPPOS com o\ncomando WRITE_HEADER porque o ACS já recebeu a sequência de\nposições da lâmina."
          n957 = flat-sequence {
            tunnel: w2582 -> [w2609]
            tunnel: [w2609] -> w2581
            frame #0 {
              n958 = Tick Count (ms)() -> (millisecond timer value=w2608:u32)
              "time 2" <- w2608
              n959 = local read "time1"() -> (w2607:u32)
              n960 = Subtract(x=w2608, y=w2607) -> (x-y=→"delay wp":u32)
            }
          }
          n961 = call "Read Instrument.lvclass.vi"("error in (no error)"=w2581, "S4ACS_GUI in"=w2589) -> ("error out"=w2594:errorcluster, "Instrument.lvclass"=w2595:refnum<class "Instrument.lvclass">, "S4ACS_GUI out"=w2591:refnum<class "S4GUI.lvclass">)  [unwired: 7 in]
          n962 = call "Read WPROT.vi"("error in (no error)"=w2594, "Instrument in"=w2595) -> ("error out"=w2588:errorcluster, "Opt_Selector.lvclass"=w2587:refnum<class "Opt_Selector.lvclass">, "Instrument out"=w2593:refnum<class "Instrument.lvclass">)  [unwired: 7 in]
          n963 = call-dynamic "Read State Machine.vi"("error in (no error)"=w2588, "Device in"=w2587) -> ("error out"=w2566:errorcluster, "State Machine.lvclass"=w2569:refnum<class "State Machine.lvclass">, "Device out"=w2585:refnum<class "Opt_Selector.lvclass">)  [unwired: 7 in]
          n964 = call-dynamic "Verif Clock 2.vi"("error in (no error)"=w2566, "period (ms)"=u32 20000 ("period"), "State Machine in"=w2569) -> ("error out"=w2565:errorcluster, "time elapsed"=→"time elapsed":u32, "State Machine out"=w2568:refnum<class "State Machine.lvclass">)  [unwired: 6 in]
          n965 = call-dynamic "Read Timeout 2.vi"("error in (no error)"=w2565, "State Machine in"=w2568) -> ("error out"=w2564:errorcluster, "Timeout 2"=w2570:bool, "State Machine out"=w2567:refnum<class "State Machine.lvclass">)  [unwired: 7 in]
          n966 = call-dynamic "Read State.vi"("error in (no error)"=w2564, "State Machine in"=w2567) -> ("error out"=w2579:errorcluster, "State"=w2583:i32, "State Machine out"=w2580:refnum<class "State Machine.lvclass">)  [unwired: 7 in]
          n967 = Equal To 0?(x=w2583) -> (x = 0?=w2557:bool)
          n968 = call-dynamic "Write State Machine.vi"("error in (no error)"=w2579, "State Machine.lvclass"=w2580, "Device in"=w2585) -> ("error out"=w2584:errorcluster, "Device out"=w2586:refnum<class "Opt_Selector.lvclass">)  [unwired: 7 in]
          n969 = call "Write WPROT.vi"("error in (no error)"=w2584, "Opt_Selector.lvclass"=w2586, "Instrument in"=w2593) -> ("error out"=w2590:errorcluster, "Instrument out"=w2592:refnum<class "Instrument.lvclass">)  [unwired: 7 in]
          n970 = call "Write Instrument.lvclass.vi"("error in (no error)"=w2590, "Instrument.lvclass"=w2592, "S4ACS_GUI in"=w2591) -> ("error out"=w2572:errorcluster, "S4ACS_GUI out"=w2563:refnum<class "S4GUI.lvclass">)  [unwired: 7 in]
          n971 = case shown="True" w2570 {
            tunnel: w2558 -> [w2598 _]
            tunnel: [w2598 u32 1 ("Obs_state")] -> w2559
            tunnel: w2563 -> [w2597 w2603]
            tunnel: [w2597 w2602] -> w2562
            tunnel: [w2596 FALSE] -> w2556
            tunnel: w2557 -> [w2596 _]
            frame False {
            }
            frame True {
              n972 = Bundle By Name(cluster=w2603, "Error Msg"="ERROR: moving waveplate timeout  (S4GUI:HandleObservationSync.vi - state 302)") -> (w2602:refnum<class "S4GUI.lvclass">)
            }
          }
          n973 = Unbundle By Name(w2563) -> ("cyclesDone"=w2576:u32, "seqAtual"=w2575:u32)
          n974 = Decrement(x=w2575) -> (x-1=w2560:u32)
          n975 = Add(x=w2576, y=w2560) -> (x+y=w2574:u32)
          n976 = Equal To 0?(x=w2574) -> (x = 0?=w2577:bool)
          n977 = Increment(x=w2558) -> ()  [unwired: 1 out]
          n978 = case shown="True" w2577 {
            tunnel: [u32 308 ("t") u32 308 ("t")] -> w2555
            frame False {
              (unwired) u32 310 ("t")
              # "Não é 1a seq:\nvai direto para\nenvio do trigger"
            }
            frame True {
              # "1a sequencia:\nenvia EXPOSE"
            }
          }
          n979 = Select(t=w2555, s=w2556, f=w2559) -> (s? t:f=w2578:u32)
          n980 = Bundle By Name(cluster=w2562, "Obs_state"=w2578) -> (w2573:refnum<class "S4GUI.lvclass">)
        }
        frame 305 {
          # "Pausa de 200ms entre o posicionamento da \nlâmina e o envio de EXPOSE para o ACS."
          n981 = flat-sequence {
            tunnel: w2621 -> [w2628]
            tunnel: [w2628] -> w2613
            frame #0 {
              n982 = Tick Count (ms)() -> (millisecond timer value=w2626:u32)
              n983 = local read "time1"() -> (w2627:u32)
              n984 = Subtract(x=w2626, y=w2627) -> (x-y=w2625:u32)
              n985 = local write "delay wp"(w2625) -> ()
            }
          }
          n986 = Tick Count (ms)() -> (millisecond timer value=w2610:u32)
          n987 = local read "time 2"() -> (w2616:u32)
          n988 = Subtract(x=w2610, y=w2616) -> (x-y=w2618:u32)
          n989 = To Double Precision Float(number=w2618) -> (double precision float=w2619:dbl)
          n990 = Less?(x=200.0 ("y"), y=w2619) -> (x < y?=w2615:bool)
          n991 = case shown="True" w2615 {
            tunnel: [w2622 u32 308 ("t")] -> w2612
            tunnel: w2611 -> [w2622 _]
            tunnel: w2610 -> [_ w2623]
            frame False {
            }
            frame True {
              # "1a sequencia:\nenvia EXPOSE"
              n992 = local write "time 2"(w2623) -> ()
            }
          }
          n993 = Bundle By Name(cluster=w2614, "Obs_state"=w2612) -> (w2620:refnum<class "S4GUI.lvclass">)
        }
        frame 308 {
          n994 = call-dynamic "Read AcquisitionA.vi"("error in (no error)"=w2691, "S4ACS_GUI in"=w2692) -> ("error out"=w2646:errorcluster, "Acquisition.lvclass"=w2647:refnum<class "Acquisition.lvclass">, "S4ACS_GUI out"=w2694:refnum<class "S4GUI.lvclass">)  [unwired: 7 in]
          n995 = call-dynamic "Read enabled.vi"("error in (no error)"=w2646, "Server in"=w2647) -> ("error out"=w2645:errorcluster, "enabled"=w2632:bool, "Server out"=w2648:refnum<class "Acquisition.lvclass">)  [unwired: 7 in]
          n996 = call "Read connection.vi"("error in (no error)"=w2645, "Server in"=w2648) -> ("error out"=w2671:errorcluster, "connection"=w2655:bool, "Server out"=w2672:refnum<class "Acquisition.lvclass">)  [unwired: 7 in]
          n997 = And(x=w2655, y=w2632) -> (x .and. y?=w2656:bool)
          n998 = case shown="True" w2656 {
            tunnel: w2672 -> [w2801 w2817]
            tunnel: w2671 -> [w2800 w2816]
            tunnel: [w2801 w2814] -> w2695
            tunnel: [w2800 w2813] -> w2693
            tunnel: [w2797 u32 0 ("New_State")] -> w2661
            tunnel: w2632 -> [w2796 _]
            frame False {
              n999 = Select(t=u32 1, s=w2796, f=u32 0) -> (s? t:f=w2797:u32)
            }
            frame True {
              n1000 = call-dynamic "Read Channel.vi"("error in (no error)"=w2816, "Acquisition in"=w2817) -> ("error out"=w2809:errorcluster, "Channel.lvclass"=w2808:refnum<class "Channel.lvclass">, "Acquisition out"=w2815:refnum<class "Acquisition.lvclass">)  [unwired: 7 in]
              n1001 = call-dynamic "Read State Machine.vi"("error in (no error)"=w2809, "Device in"=w2808) -> ("error out"=w2810:errorcluster, "State Machine.lvclass"=w2812:refnum<class "State Machine.lvclass">, "Device out"=w2806:refnum<class "Channel.lvclass">)  [unwired: 7 in]
              n1002 = call "Next State.vi"("error in (no error)"=w2810, "New_State"=50, "State Machine in"=w2812) -> ("error out"=w2803:errorcluster, "State Machine out"=w2804:refnum<class "State Machine.lvclass">)  [unwired: 7 in]
              n1003 = call-dynamic "Write State Machine.vi"("error in (no error)"=w2803, "State Machine.lvclass"=w2804, "Device in"=w2806) -> ("error out"=w2805:errorcluster, "Device out"=w2807:refnum<class "Channel.lvclass">)  [unwired: 7 in]
              n1004 = call-dynamic "Write Channel.vi"("error in (no error)"=w2805, "Channel.lvclass"=w2807, "Acquisition in"=w2815) -> ("error out"=w2813:errorcluster, "Acquisition out"=w2814:refnum<class "Acquisition.lvclass">)  [unwired: 7 in]
            }
          }
          n1005 = call-dynamic "Write AcquisitionA.vi"("error in (no error)"=w2693, "Acquisition.lvclass"=w2695, "S4ACS_GUI in"=w2694) -> ("error out"=w2688:errorcluster, "S4ACS_GUI out"=w2689:refnum<class "S4GUI.lvclass">)  [unwired: 7 in]
          n1006 = call "Read AcquisitionB.vi"("error in (no error)"=w2688, "S4ACS_GUI in"=w2689) -> ("error out"=w2642:errorcluster, "Acquisition.lvclass"=w2644:refnum<class "Acquisition.lvclass">, "S4ACS_GUI out"=w2686:refnum<class "S4GUI.lvclass">)  [unwired: 7 in]
          n1007 = call-dynamic "Read enabled.vi"("error in (no error)"=w2642, "Server in"=w2644) -> ("error out"=w2641:errorcluster, "enabled"=w2631:bool, "Server out"=w2643:refnum<class "Acquisition.lvclass">)  [unwired: 7 in]
          n1008 = call "Read connection.vi"("error in (no error)"=w2641, "Server in"=w2643) -> ("error out"=w2669:errorcluster, "connection"=w2653:bool, "Server out"=w2670:refnum<class "Acquisition.lvclass">)  [unwired: 7 in]
          n1009 = And(x=w2653, y=w2631) -> (x .and. y?=w2654:bool)
          n1010 = case shown="True" w2654 {
            tunnel: w2670 -> [w2779 w2795]
            tunnel: w2669 -> [w2778 w2794]
            tunnel: [w2779 w2792] -> w2687
            tunnel: [w2778 w2791] -> w2685
            tunnel: [w2775 u32 0 ("New_State")] -> w2660
            tunnel: w2631 -> [w2774 _]
            frame False {
              n1011 = Select(t=u32 2, s=w2774, f=u32 0) -> (s? t:f=w2775:u32)
            }
            frame True {
              n1012 = call-dynamic "Read Channel.vi"("error in (no error)"=w2794, "Acquisition in"=w2795) -> ("error out"=w2787:errorcluster, "Channel.lvclass"=w2786:refnum<class "Channel.lvclass">, "Acquisition out"=w2793:refnum<class "Acquisition.lvclass">)  [unwired: 7 in]
              n1013 = call-dynamic "Read State Machine.vi"("error in (no error)"=w2787, "Device in"=w2786) -> ("error out"=w2788:errorcluster, "State Machine.lvclass"=w2790:refnum<class "State Machine.lvclass">, "Device out"=w2784:refnum<class "Channel.lvclass">)  [unwired: 7 in]
              n1014 = call "Next State.vi"("error in (no error)"=w2788, "New_State"=50, "State Machine in"=w2790) -> ("error out"=w2781:errorcluster, "State Machine out"=w2782:refnum<class "State Machine.lvclass">)  [unwired: 7 in]
              n1015 = call-dynamic "Write State Machine.vi"("error in (no error)"=w2781, "State Machine.lvclass"=w2782, "Device in"=w2784) -> ("error out"=w2783:errorcluster, "Device out"=w2785:refnum<class "Channel.lvclass">)  [unwired: 7 in]
              n1016 = call-dynamic "Write Channel.vi"("error in (no error)"=w2783, "Channel.lvclass"=w2785, "Acquisition in"=w2793) -> ("error out"=w2791:errorcluster, "Acquisition out"=w2792:refnum<class "Acquisition.lvclass">)  [unwired: 7 in]
            }
          }
          n1017 = call "Write AcquisitionB.vi"("error in (no error)"=w2685, "Acquisition.lvclass"=w2687, "S4ACS_GUI in"=w2686) -> ("error out"=w2681:errorcluster, "S4ACS_GUI out"=w2680:refnum<class "S4GUI.lvclass">)  [unwired: 7 in]
          n1018 = call-dynamic "Read AcquisitionC.vi"("error in (no error)"=w2681, "S4ACS_GUI in"=w2680) -> ("error out"=w2638:errorcluster, "Acquisition.lvclass"=w2640:refnum<class "Acquisition.lvclass">, "S4ACS_GUI out"=w2683:refnum<class "S4GUI.lvclass">)  [unwired: 7 in]
          n1019 = call-dynamic "Read enabled.vi"("error in (no error)"=w2638, "Server in"=w2640) -> ("error out"=w2637:errorcluster, "enabled"=w2630:bool, "Server out"=w2639:refnum<class "Acquisition.lvclass">)  [unwired: 7 in]
          n1020 = call "Read connection.vi"("error in (no error)"=w2637, "Server in"=w2639) -> ("error out"=w2667:errorcluster, "connection"=w2650:bool, "Server out"=w2668:refnum<class "Acquisition.lvclass">)  [unwired: 7 in]
          n1021 = And(x=w2650, y=w2630) -> (x .and. y?=w2652:bool)
          n1022 = case shown="True" w2652 {
            tunnel: [w2756 w2765] -> w2684
            tunnel: [w2757 w2764] -> w2682
            tunnel: w2668 -> [w2757 w2762]
            tunnel: w2667 -> [w2756 w2761]
            tunnel: [w2753 u32 0 ("New_State")] -> w2659
            tunnel: w2630 -> [w2752 _]
            frame False {
              n1023 = Select(t=u32 4, s=w2752, f=u32 0) -> (s? t:f=w2753:u32)
            }
            frame True {
